vi "dvp Vi Get Saturation.vi"(10 "pSaturation":i32, 11 "handle":u32) -> (2 "pSaturation out":i32, 3 "function return":u32(ring))   [LabVIEW 2018, in "LabViewDVPCamera.lvlib"]
doc: "LabviewDvp2Api dvpStatus dvpViGetSaturation(dvpHandle handle, dvpInt32 *pSaturation);"
uses:
  LabViewDVPCamera.lvlib
  LabViewDVPCamera/LabViewDVPCamera.dll
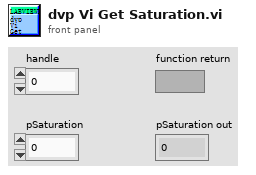
[diagram p1: front panel]
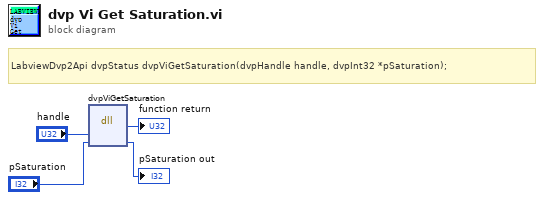
[diagram p0: block diagram]
diagram:
  # "LabviewDvp2Api dvpStatus dvpViGetSaturation(dvpHandle handle, dvpInt32 *pSaturation);"
  n1 = dll-call lib="C:/Program Files (x86)/DVP2 Labview cn 64/Sample/LabViewDVPCamera/LabViewDVPCamera.*" fn="dvpViGetSaturation"("handle"="handle", "pSaturation"="pSaturation") -> (→"function return":u32, "pSaturation"=→"pSaturation out":i32)  [unwired: 4 in, 2 out]
